vi "RSZVB Configure Loss.vi"(5 "Loss At DC (0.0 dB)":dbl format="%^.3e", 6 "Loss Reference Frequency (1.0e+9 Hz)":dbl=1000000000.0 format="%^.3e", 7 "Loss At Frequency (0.0 dB)":dbl format="%^.3e", 8 "error in (no error)":errorcluster {"code" format="%.0x"}, 9 "Port (1)":i32=1, 10 "Channel (1)":i32=1, 11 "VISA session":refnum<visa-resource-name>) -> (0 "error out":errorcluster {"code" format="%.0x"}, 3 "dup VISA session":refnum<visa-resource-name>)   [LabVIEW 2011]
doc: "This VI configures parameters of One-way Loss.\n\nRemote-control command(s):\n[SENSe<Ch>:]CORRection:LOSS<port_no> <DC_loss>\n[SENSe<Ch>:]CORRection:LOSS<port_no>:OFFSet <ref_loss>\n[SENSe<Ch>:]CORRection:LOSS<port_no>:FREQuency <ref_frequency>"
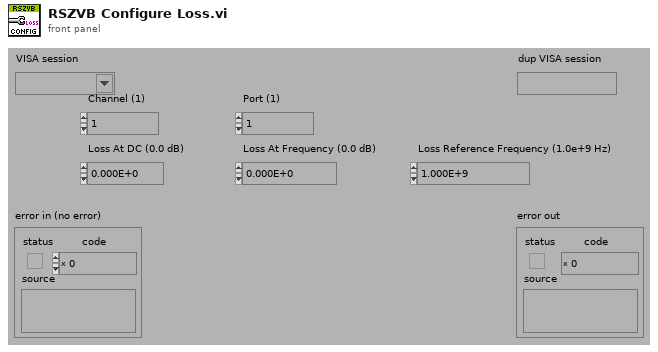
[diagram p1: front panel]
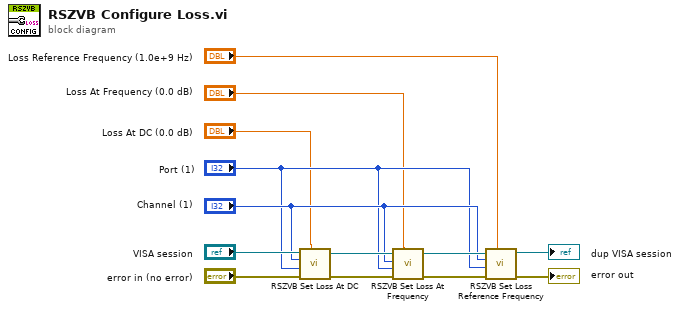
[diagram p0: block diagram]
diagram:
  n1 = call "RSZVB Set Loss At DC.vi"("Loss At DC (0.0 dB)"="Loss At DC (0.0 dB)", "error in (no error)"="error in (no error)", "Port (1)"="Port (1)", "Channel (1)"="Channel (1)", "VISA session"="VISA session") -> ("error out"=w8:errorcluster, "dup VISA session"=w12:refnum<visa-resource-name>)  [unwired: 5 in]
  n2 = call "RSZVB Set Loss At Frequency.vi"("Loss At Frequency (0.0 dB)"="Loss At Frequency (0.0 dB)", "error in (no error)"=w8, "Port (1)"="Port (1)", "Channel (1)"="Channel (1)", "VISA session"=w12) -> ("error out"=w7:errorcluster, "dup VISA session"=w11:refnum<visa-resource-name>)  [unwired: 5 in]
  n3 = call "RSZVB Set Loss Reference Frequency.vi"("Loss Reference Frequency (1.0e+9 Hz)"="Loss Reference Frequency (1.0e+9 Hz)", "error in (no error)"=w7, "Port (1)"="Port (1)", "Channel (1)"="Channel (1)", "VISA session"=w11) -> ("error out"=→"error out":errorcluster, "dup VISA session"=→"dup VISA session":refnum<visa-resource-name>)  [unwired: 5 in]
